vi "SPT-Create Envelope.vi"(0 "SPT.Properties":T1, 7 "Fs (Hz)":dbl, 11 "error in (no error)":errorcluster) -> (8 "Env":dbl[](array[numeric]), 15 "error out":errorcluster)   [LabVIEW 2015]
uses:
  SPT-Properties.ctl
  SPT-Shape.ctl
  Utility VIs/Math VIs/LinSpace (x0-dx-npts).vi
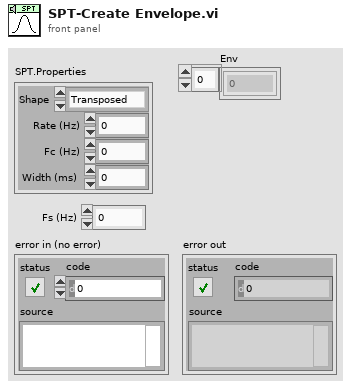
[diagram p1: front panel]
types:
  T1 = typedef "SPT-Properties.ctl" = cluster{"Shape":T2, "Rate (Hz)":dbl, "Fc (Hz)":dbl, "Width (ms)":dbl}
  T2 = typedef "SPT-Shape.ctl" = enum16{"Transposed", "Alpha", "Gabor"}
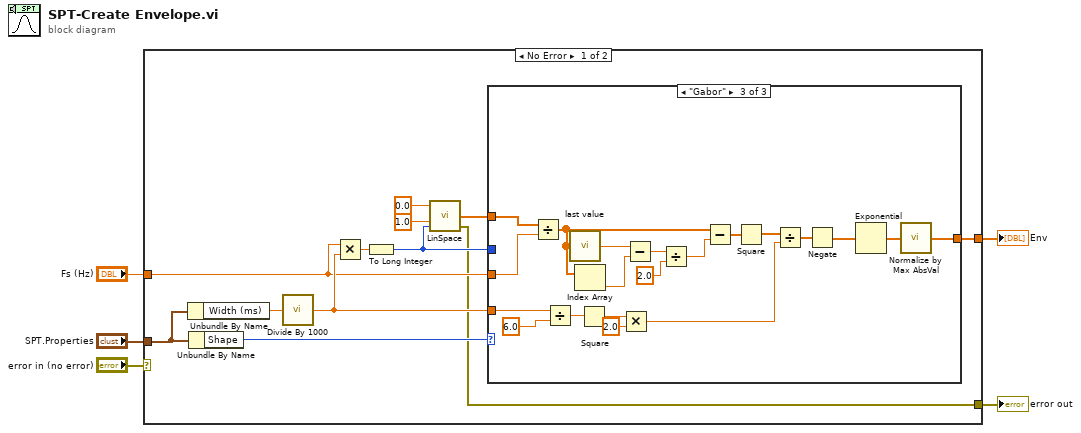
[diagram p0: block diagram]
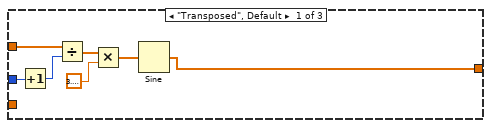
[diagram p2: hidden frame]
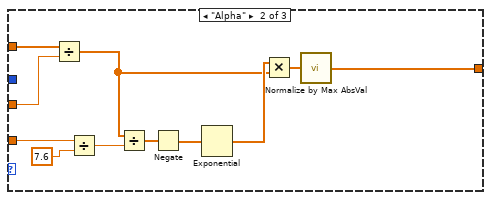
[diagram p3: hidden frame]
diagram:
  n1 = case shown="No Error" "error in (no error)" {
    selector: "error in (no error)" -> [_ w56]
    tunnel: "SPT.Properties" -> [w12 _]
    tunnel: "Fs (Hz)" -> [w8 _]
    tunnel: [w7 _] -> w3
    tunnel: [w6 w56] -> w1
    frame No Error {
      n2 = Unbundle By Name(w12) -> ("Width (ms)"=w17:dbl)
      n3 = Unbundle By Name(w12) -> ("Shape"=w11:T2)
      n4 = call "Divide By 1000.vi"("X"=w17) -> ("X/1000"=w9:dbl)
      n5 = Multiply(x=w8, y=w9) -> (x*y=w16:dbl)
      n6 = To Long Integer(number=w16) -> (32bit integer=w10:i32)
      n7 = call-poly "LinSpace.vi"("npts"=w10, "dx"=1.0, "x0"=0.0) -> ("error out"=w6:errorcluster, "Array"=w13:dbl[])  [unwired: 1 in]
      n8 = case shown="\"Gabor\"" w11 {
        tunnel: w13 -> [w24 w33 w53]
        tunnel: w10 -> [w23 _ _]
        tunnel: w9 -> [_ w35 w55]
        tunnel: w8 -> [_ w32 w52]
        tunnel: [w18 w25 w36] -> w7
        frame "Transposed", Default {
          n9 = Increment(x=w23) -> (x+1=w22:i32)
          n10 = Divide(x=w24, y=w22) -> (x/y=w21:dbl[])
          n11 = Multiply(x=w21, y=3.141592653589793) -> (x*y=w19:dbl[])
          n12 = Sine(x=w19) -> (sin(x)=w18:dbl[])
        }
        frame "Alpha" {
          n13 = Divide(x=w33, y=w32) -> (x/y=w27:dbl[])
          n14 = Divide(x=w35, y=7.6) -> (x/y=w31:dbl)
          n15 = Divide(x=w27, y=w31) -> (x/y=w30:dbl[])
          n16 = Negate(x=w30) -> (-x=w29:dbl[])
          n17 = Exponential(1:w29) -> (0:w28:dbl[])
          n18 = Multiply(x=w28, y=w27) -> (x*y=w26:dbl[])
          n19 = call "Normalize by Max AbsVal.vi"("Y"=w26) -> ("Ynorm"=w25:dbl[])
        }
        frame "Gabor" {
          n20 = Divide(x=w53, y=w52) -> (x/y=w44:dbl[])
          n21 = Divide(x=w55, y=6.0) -> (x/y=w42:dbl)
          n22 = call "last value.vi"("array"=w44) -> ("element"=w48:dbl)
          n23 = Index Array(array=w44) -> (element=w49:dbl)  [unwired: 1 in]
          n24 = Square(x=w42) -> (x^2=w41:dbl)
          n25 = Multiply(x=w41, y=2.0) -> (x*y=w38:dbl)
          n26 = Subtract(x=w48, y=w49) -> (x-y=w47:dbl)
          n27 = Divide(x=w47, y=2.0) -> (x/y=w45:dbl)
          n28 = Subtract(x=w44, y=w45) -> (x-y=w43:dbl[])
          n29 = Square(x=w43) -> (x^2=w39:dbl[])
          n30 = Divide(x=w39, y=w38) -> (x/y=w37:dbl[])
          n31 = Negate(x=w37) -> (-x=w51:dbl[])
          n32 = Exponential(1:w51) -> (0:w50:dbl[])
          n33 = call "Normalize by Max AbsVal.vi"("Y"=w50) -> ("Ynorm"=w36:dbl[])
        }
      }
    }
    frame Error {
    }
  }
  "error out" <- w1
  "Env" <- w3
